vi "Create Slots.vi"(7 "error in":errorcluster, 8 "EtherCAT?":bool, 9 "Num Slots":i32=8, 10 "Item Ref In":T1 format="%.0x") -> (0 "error out":errorcluster, 3 "Item Ref out":T1 format="%.0x")   [LabVIEW 2017, in "Scan Engine Custom Device.lvlib"]
uses:
  Scan Engine Custom Device.lvlib
  <vilib>/NI Veristand/Custom Device API/Custom Device API.lvlib
  Globals/Property Strings.vi
  Modules.lvlibp/RSI Module/Module Models.ctl
  Modules.lvlibp/RSI Module/Slot Settings.ctl
  Globals/Scan Engine GUIDs.vi
  Globals/String Constants.vi
  Modules.lvlibp/RSI Module/Class Property Strings.vi
  <vilib>/NI Veristand/Custom Device API/Custom Device Item Ref.ctl
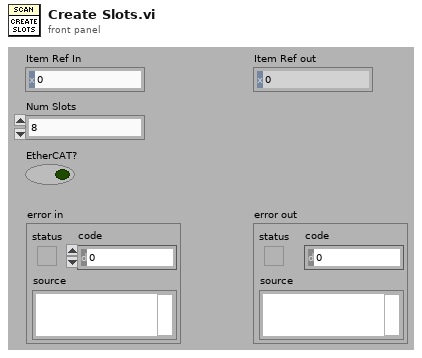
[diagram p1: front panel]
types:
  T1 = typedef "Custom Device API.lvlib/Custom Device Item Ref.ctl" = u64
  T2 = typedef "Modules.lvlibp/RSI Module.lvclass/Slot Settings.ctl" = cluster{"Slot":u32, "EtherCAT?":bool}
  T3 = typedef "Modules.lvlibp/RSI Module.lvclass/Module Models.ctl" = enum16{"Empty", "NI 9201", "NI 9203", "NI 9205", "NI 9206", "NI 9207", "NI 9208", "NI 9211", "NI 9212", "NI 9213", "NI 9214", "NI 9215", "NI 9217", "NI 9219", "NI 9220", "NI 9221", "NI 9222", "NI 9223", "NI 9225", "NI 9227", "NI 9229", "NI 9233", "NI 9234", "NI 9235", "NI 9236", "NI 9237", "NI 9239", "NI 9242", "NI 9244", "NI 9263", "NI 9264", "NI 9265", "NI 9269", "NI 9375", "NI 9401", "NI 9402", "NI 9403", "NI 9411", "NI 9421", "NI 9422", "NI 9423", "NI 9425", "NI 9426", "NI 9435", "NI 9437", "NI 9472", "NI 9474", "NI 9475", "NI 9476", "NI 9477", "NI 9478", "NI 9481", "NI 9482", "NI 9485"}
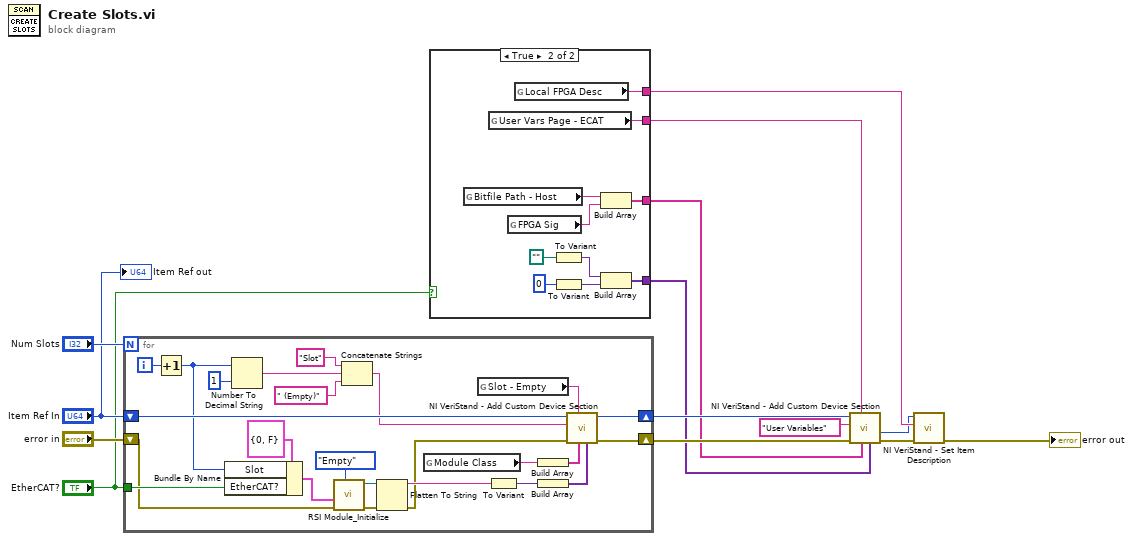
[diagram p0: block diagram]
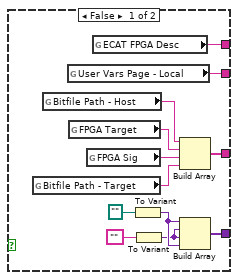
[diagram p2: hidden frame]
diagram:
  n1 = for {
    N: "Num Slots" -> [_]
    tunnel: "EtherCAT?" -> [w24]
    shift-right: [w33] -> w11
    shift-left: "error in" -> [w20]
    shift-right: [w32] -> w12
    shift-left: "Item Ref In" -> [w38]
    i -> [w35]
    n2 = Increment(x=w35) -> (x+1=w29:i32)
    n3 = Bundle By Name(cluster=T2 {"Slot"=0, "EtherCAT?"=FALSE} ("Slot Settings"), "Slot"=w29, "EtherCAT?"=w24) -> (w18:T2)
    n4 = Number To Decimal String(number=w29, width (-)=i16 1) -> (decimal integer string=w37:string)
    n5 = call "RSI Module_Initialize.vi"("Module Model"=Module_Models."Empty" ("Module"), "error in (no error)"=w20, "Slot Settings"=w18) -> ("error out"=w19:errorcluster, "RSI Module out"=w15:refnum<class "RSI Module.lvclass">)  [unwired: 7 in]
    n6 = Concatenate Strings("Slot" ("string"), w37, " (Empty)" ("Section Name")) -> (w34:string)
    n7 = Flatten To String(anything=w15, error in (no error)=w19) -> (data string=w23:string, error out=w22:errorcluster)  [unwired: 2 in, 1 out]
    n8 = global read "Class Property Strings.vi" "Module Class"() -> (w21:string)
    n9 = global read "Scan Engine GUIDs.vi" "Slot - Empty"() -> (w25:string)
    n10 = To Variant(anything=w23) -> (Variant=w30:variant)
    n11 = Build Array(w21) -> (w27:string[])
    n12 = Build Array(w30) -> (w31:variant[])
    n13 = call <vilib>:"NI VeriStand - Add Custom Device Section.vi"("Property Values"=w31, "Property names"=w27, "GUID (Default Section)"=w25, "error in (no error)"=w22, "Section Name"=w34, "Parent Ref in"=w38) -> ("error out"=w33:errorcluster, "Parent Ref out"=w32:T1)  [unwired: 2 in, 2 out]
  }
  n14 = case shown="True" "EtherCAT?" {
    tunnel: [w42 w52] -> w8
    tunnel: [w41 w53] -> w7
    tunnel: [w40 w54] -> w9
    tunnel: [w39 w51] -> w4
    frame False {
      n15 = global read "Property Strings.vi" "Bitfile Path - Target"() -> (w46:string)
      n16 = global read "Property Strings.vi" "Bitfile Path - Host"() -> (w49:string)
      n17 = global read "Scan Engine GUIDs.vi" "User Vars Page - Local"() -> (w40:string)
      n18 = global read "Property Strings.vi" "FPGA Target"() -> (w48:string)
      n19 = global read "Property Strings.vi" "FPGA Sig"() -> (w47:string)
      n20 = global read "String Constants.vi" "ECAT FPGA Desc"() -> (w39:string)
      n21 = To Variant(anything=path "") -> (Variant=w45:variant)
      n22 = To Variant(anything="") -> (Variant=w43:variant)
      n23 = Build Array(w49, w48, w47, w46) -> (w41:string[])
      n24 = Build Array(w45, w43, w43, w45) -> (w42:variant[])
    }
    frame True {
      n25 = global read "Property Strings.vi" "Bitfile Path - Host"() -> (w56:string)
      n26 = global read "Scan Engine GUIDs.vi" "User Vars Page - ECAT"() -> (w54:string)
      n27 = global read "Property Strings.vi" "FPGA Sig"() -> (w55:string)
      n28 = global read "String Constants.vi" "Local FPGA Desc"() -> (w51:string)
      n29 = To Variant(anything=path "") -> (Variant=w58:variant)
      n30 = To Variant(anything=u32 0 ("ModuleIdent (ECAT)")) -> (Variant=w57:variant)
      n31 = Build Array(w56, w55) -> (w53:string[])
      n32 = Build Array(w58, w57) -> (w52:variant[])
    }
  }
  n33 = call <vilib>:"NI VeriStand - Add Custom Device Section.vi"("Property Values"=w8, "Property names"=w7, "GUID (Default Section)"=w9, "error in (no error)"=w11, "Section Name"="User Variables", "Parent Ref in"=w12) -> ("error out"=w3:errorcluster, "Section Ptr"=w2:T1)  [unwired: 2 in, 2 out]
  n34 = call <vilib>:"NI VeriStand - Set Item Description.vi"("error in (no error)"=w3, "Description"=w4, "Item Ref in"=w2) -> ("error out"=→"error out":errorcluster)  [unwired: 6 in, 2 out]
  "Item Ref out" <- "Item Ref In"
